vi "Obtain Queue with Initialize.vi"(8 "Error In":errorcluster, 11 "Queue Name":string) -> (0 "Error Out":errorcluster, 3 "Queue out":refnum<queue>)   [LabVIEW 2019, in "Queues.lvlib"]
uses:
  Queues.lvlib
  Message Cluster.ctl
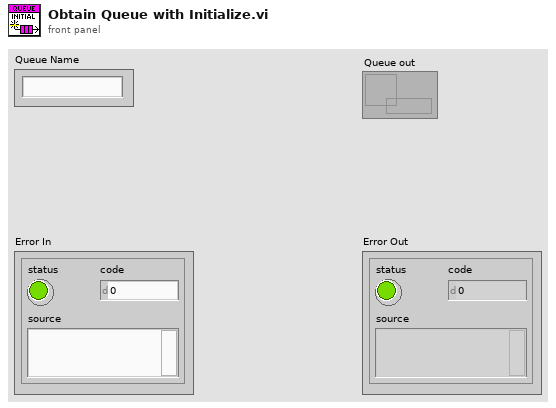
[diagram p1: front panel]
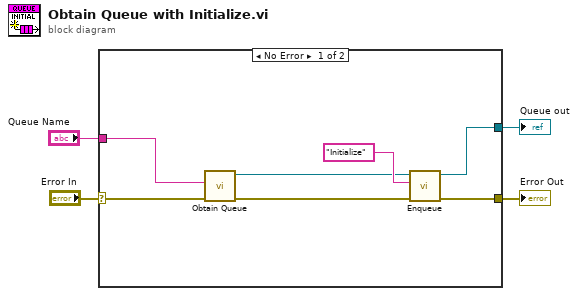
[diagram p0: block diagram]
diagram:
  n1 = case shown="No Error" "Error In" {
    selector: "Error In" -> [w8 w12]
    tunnel: [w10 w12] -> w4
    tunnel: [w9 _] -> w2
    tunnel: "Queue Name" -> [w5 _]
    frame No Error {
      n2 = call "Obtain Queue.vi"("Error In"=w8, "Queue Name"=w5) -> ("Error Out"=w7:errorcluster, "queue out"=w6:refnum<queue>)  [unwired: 8 in]
      n3 = call "Enqueue.vi"("Error In"=w7, "State"="Initialize", "Queue in"=w6) -> ("Error Out"=w10:errorcluster, "Queue out"=w9:refnum<queue>)  [unwired: 7 in]
    }
    frame Error {
    }
  }
  "Error Out" <- w4
  "Queue out" <- w2
